vi "Get Tunnel Inside Terminals.vi"(11 "Terminal in":refnum<vi>) -> (2 "Terms[0]":refnum<vi>, 3 "InsideTerms[]":refnum<vi>[](array[refnum]))   [LabVIEW 2014]
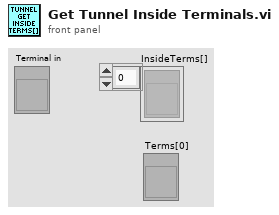
[diagram p1: front panel]
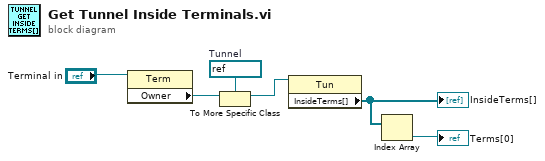
[diagram p0: block diagram]
diagram:
  w3 = refnum<vi> refnum  # Tunnel
  n1 = property on="Property Node" class="Term"(reference="Terminal in") -> ("Owner"=w5:refnum<vi>)  [unwired: 1 in, 2 out]
  n2 = To More Specific Class(target class=w3, reference=w5) -> (specific class reference=w4:refnum<vi>)  [unwired: 1 in, 1 out]
  n3 = property on="Property Node" class="Tun"(reference=w4) -> ("InsideTerms[]"=w2:refnum<vi>[])  [unwired: 1 in, 2 out]
  "InsideTerms[]" <- w2
  n4 = Index Array(array=w2) -> (element=→"Terms[0]":refnum<vi>)  [unwired: 1 in]
